vi "Find Attribute.vi"(10 "Attr Name":string, 11 "Attirbutes":T1[](array[typedef])) -> (2 "Found?":bool, 3 "Attribute Information":T1)   [LabVIEW 2020, in "Camera Settings Dialog UI.lvlib" / "Camera Settings Dialog.lvclass"]
uses:
  Camera Settings Dialog.lvclass
  Camera Settings Dialog.lvclass/Camera Settings Dialog.ctl
  Camera Attribute Info.ctl
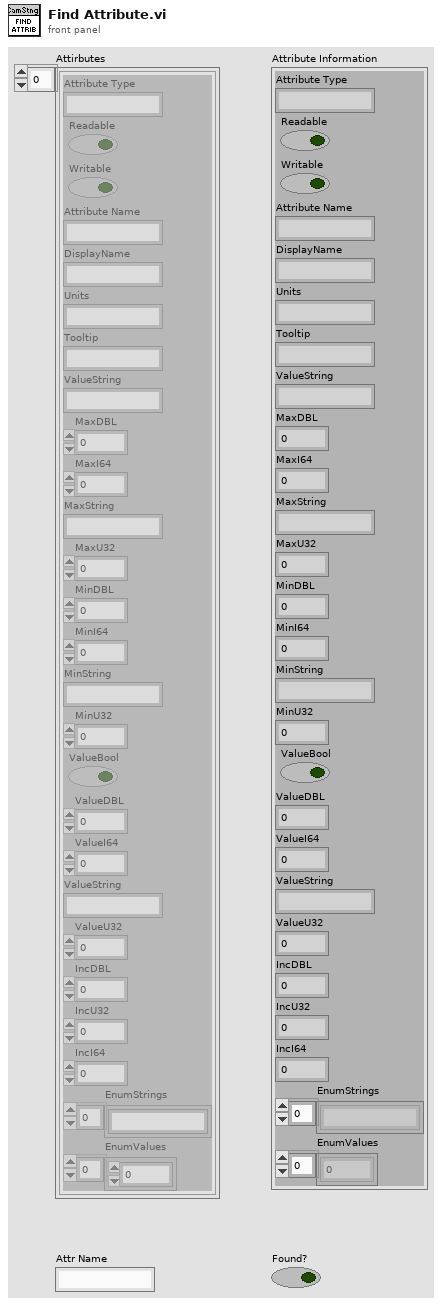
[diagram p1: front panel]
types:
  T1 = typedef "Camera Attribute Info.ctl" = cluster{"Attribute Type":string, "Readable":bool, "Writable":bool, "Attribute Name":string, "DisplayName":string, "Units":string, "Tooltip":string, "ValueString":string, "MaxDBL":dbl, "MaxI64":i64, "MaxString":string, "MaxU32":u32, "MinDBL":dbl, "MinI64":i64, "MinString":string, "MinU32":u32, "ValueBool":bool, "ValueDBL":dbl, "ValueI64 ":i64, "ValueString":string, "ValueU32":u32, "IncDBL":dbl, "IncU32":u32, "IncI64":i64, "EnumStrings":string[], "EnumValues":u32[]}
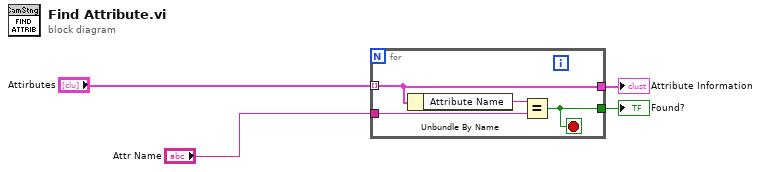
[diagram p0: block diagram]
diagram:
  n1 = for {
    tunnel: "Attirbutes" -> [w5] mode=indexing
    tunnel: "Attr Name" -> [w7]
    tunnel: [w6] -> w3
    tunnel: [w5] -> w4
    stop <- w6 stop-if-true
    n2 = Unbundle By Name(w5) -> ("Attribute Name"=w8:string)
    n3 = Equal?(x=w8, y=w7) -> (x = y?=w6:bool)
  }
  "Attribute Information" <- w4
  "Found?" <- w3
